vi "palletAnalyse.vi"() -> ()   [LabVIEW 2020, in "mainLibrary.lvlib"]
uses:
  mainLibrary.lvlib
panel:
  out "Pallet No. Sync":bool
  out "Frame False":bool
  out "Distance Sensor 3 (mm)":dbl format="%.2g"
  out "Distance Sensor 2 (mm)":dbl format="%.2g"
  out "Distance Sensor 1 (mm)":dbl format="%.2g"
  out "Right Sidewall":bool
  out "Grate-bar Defects Type":u8 format="%#.0f"
  out "Grate-bar Defects %":dbl format="%.2g"
  out "Beam Curvature (mm)":dbl format="%.2g"
  out "Left Sidewall":bool
  out "Pallet Number":u8=1 min=1 max=248 step=1 format="%03.0f"
  in  "Close":bool
  out "Pallet Image":T1(plugin-control)
  # "DPIS"
  # "Pallet Analyse"
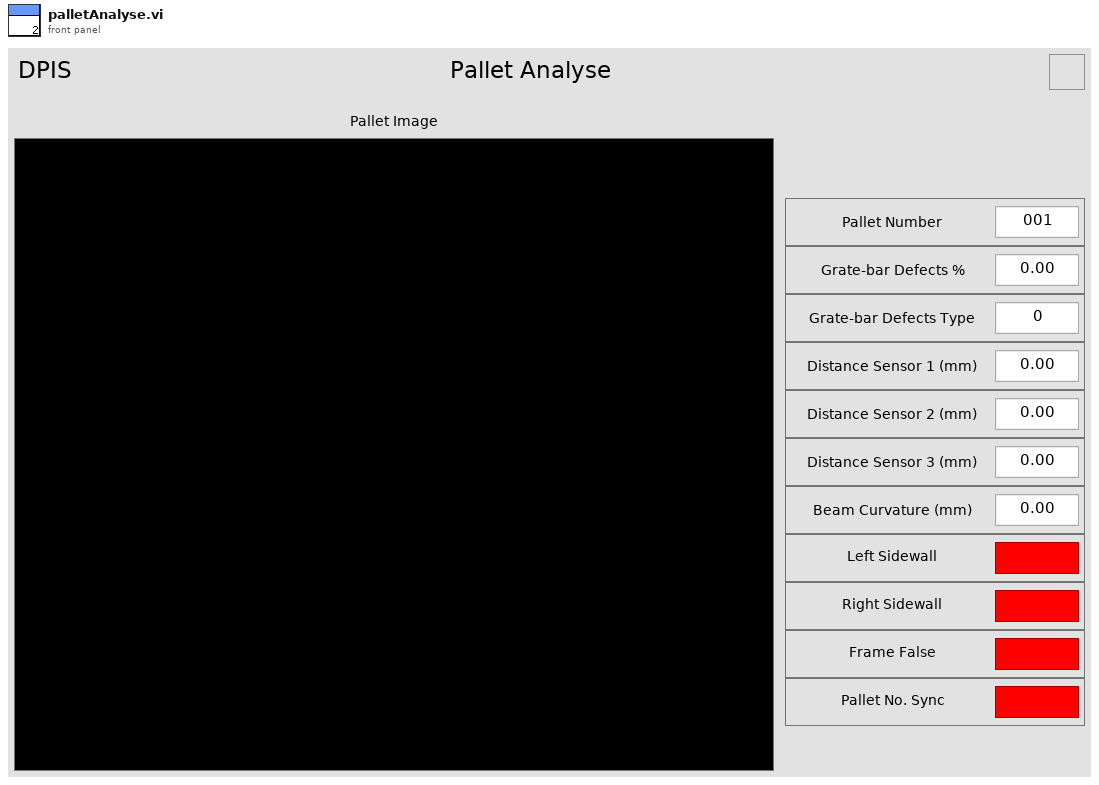
[diagram p1: front panel]
types:
  T1 = typedef "IMAQ Image.ctl" = refnum<image>
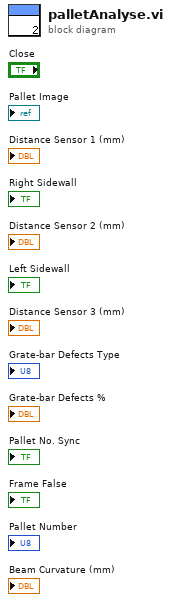
[diagram p0: block diagram]
diagram:
